vi "List Values.vi"(7 "Group":string="Default", 8 "error in (no error)":errorcluster, 9 "NI Specific Type":T2, 10 "Broad Types":T1, 11 "Blackboard in":refnum<class "Blackboard.lvclass">) -> (0 "error out":errorcluster, 1 "Values":refnum<class "Abs_Value.lvclass">[](array[class]), 2 "Tags":string[](array[string]), 3 "Blackboard out":refnum<class "Blackboard.lvclass">)   [LabVIEW 2021, in "Blackboard.lvclass"]
uses:
  Blackboard.lvclass
  <vilib>/TSA/Abstract Data Classes/Abs_Types/Value/Abs_Value.lvclass
  <vilib>/Utility/Data Type/Type Definitions/Data Type.ctl
  Support/Filter Type.ctl
  Blackboard.lvclass/Blackboard.ctl
  <vilib>/TSA/Abstract Data Classes/Abs_Types/Boolean/Abs_Boolean.lvclass
  C:/Program Files (x86)/National Instruments/LabVIEW 2021/vi.lib/TSA/Abstract Data Classes/Abs_Types/Value/Abs_Value.lvclass
  <vilib>/TSA/Abstract Data Classes/Abs_Types/String/Abs_String.lvclass
  <vilib>/TSA/Abstract Data Classes/Abs_Types/Numeric/Abs_Numeric.lvclass
  <vilib>/TSA/Abstract Data Classes/Abs_Types/Floating Point/Abs_Floating Point.lvclass
  <vilib>/TSA/Abstract Data Classes/Abs_Types/Integer/Abs_Integer.lvclass
  <vilib>/TSA/Omni-Bus/Local Bus/Support/Initialise DVR's.vi
  <vilib>/TSA/Abstract Data Classes/Abs_Types/Type/Abs_Type.lvclass
  <vilib>/Utility/Data Type/NI_Data Type.lvlib
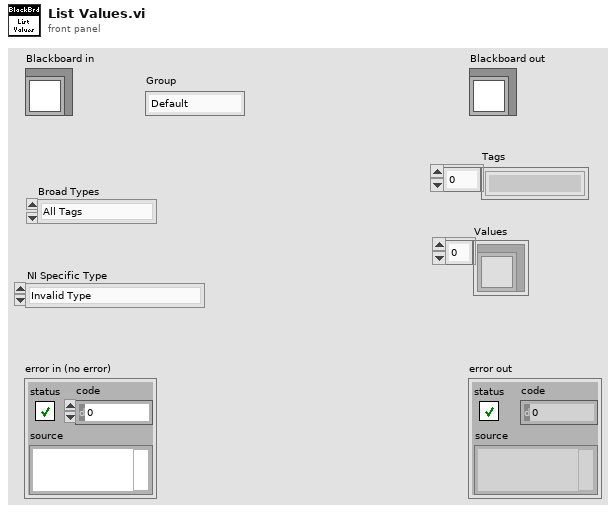
[diagram p1: front panel]
types:
  T1 = typedef "Blackboard.lvclass/Filter Type.ctl" = enum16{"All Tags", "NI Specific Type", "Boolean", "String", "Numeric", "Float", "Integer"}
  T2 = typedef "NI_Data Type.lvlib/Data Type.ctl" = enum8{"Invalid Type", "Void", "I8", "I16", "I32", "I64", "U8", "U16", "U32", "U64", "Single Float", "Double Float", "Extended Float", "Single Complex", "Double Complex", "Extended Complex", "Enum U8", "Enum U16", "Enum U32", "Enum U64", "Single Float With Unit", "Double Float With Unit", "Extended Float With Unit", "Single Complex with Unit", "Double Complex with Unit", "Extended Complex with Unit", "Boolean", "String", "Path", "Picture", "Tag", "Array", "Cluster", "Variant", "LV Variant", "Waveform", "Timestamp", "Digital Waveform", "Digital Data", "ExpressData", "Refnum", "External Data", "VI", "Poly VI", "LabVIEW Class Instance", "Fixed Point", "Set Collection", "Map Collection"}
  T3 = typedef "Blackboard.lvclass/Groups Type.ctl" = cluster{"Data":T4[], "Map":T7}
  T4 = typedef "Blackboard.lvclass/Data DVR Type.ctl" = cluster{"Tags":T5, "Data Refs":T6}
  T5 = typedef "Blackboard.lvclass/Tags Map Type.ctl" = map{string, refnum<class "Abs_Value.lvclass">}
  T6 = typedef "Local Bus.lvclass/Data Value References.ctl" = cluster{"Boolean":refnum<data-value>, "String":refnum<data-value>, "DBL":refnum<data-value>, "SGL":refnum<data-value>, "EXT":refnum<data-value>, "U8":refnum<data-value>, "U16":refnum<data-value>, "U32":refnum<data-value>, "U64":refnum<data-value>, "I8":refnum<data-value>, "I16":refnum<data-value>, "I32":refnum<data-value>, "I64":refnum<data-value>, "CDBL":refnum<data-value>, "CSGL":refnum<data-value>, "CEXT":refnum<data-value>, "Time":refnum<data-value>, "Variant":refnum<data-value>, "Waveform":refnum<data-value>, "Type":refnum<data-value>}
  T7 = typedef "Blackboard.lvclass/Group Map Type.ctl" = map{string, i32}
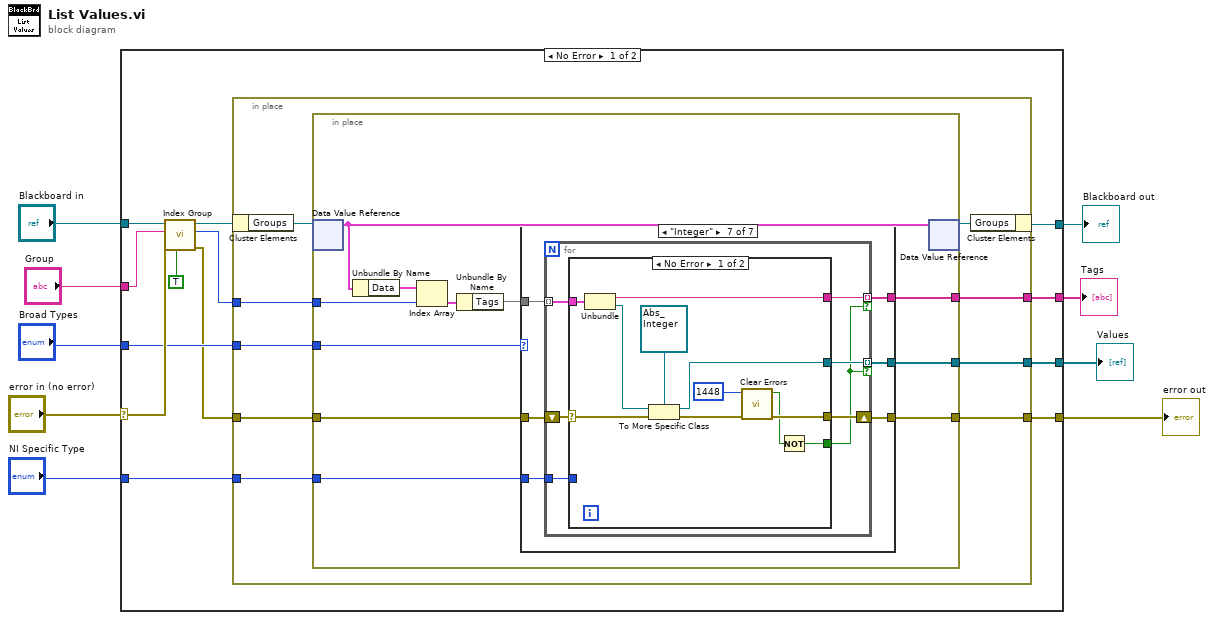
[diagram p0: block diagram]
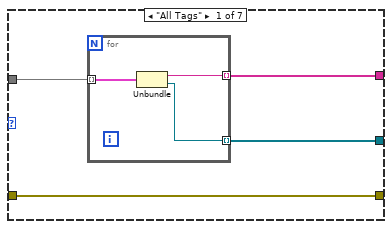
[diagram p2: hidden frame]
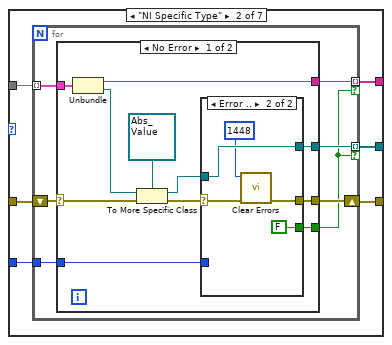
[diagram p3: hidden frame]
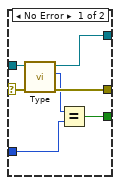
[diagram p4: hidden frame]
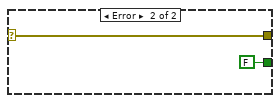
[diagram p5: hidden frame]
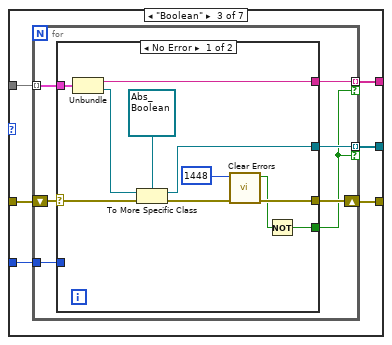
[diagram p6: hidden frame]
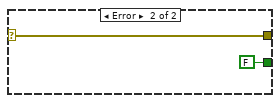
[diagram p7: hidden frame]
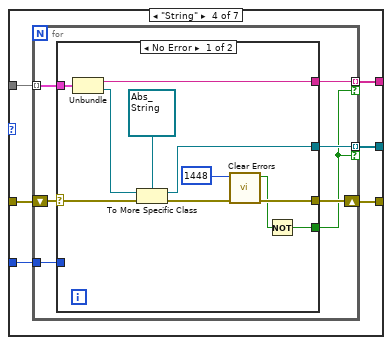
[diagram p8: hidden frame]
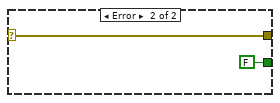
[diagram p9: hidden frame]
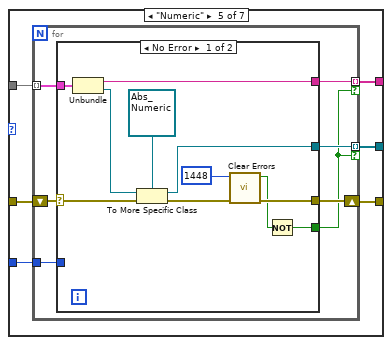
[diagram p10: hidden frame]
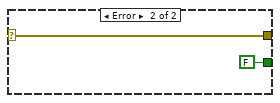
[diagram p11: hidden frame]
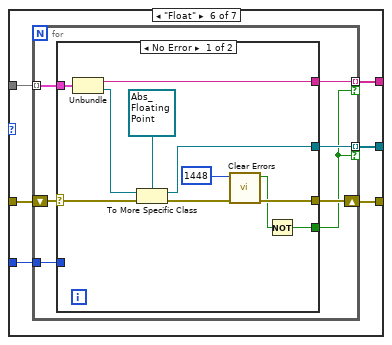
[diagram p12: hidden frame]
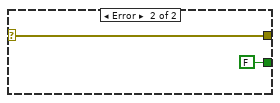
[diagram p13: hidden frame]
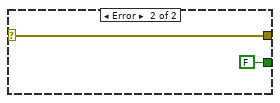
[diagram p14: hidden frame]
diagram:
  n1 = case shown="No Error" "error in (no error)" {
    selector: "error in (no error)" -> [w17 w219]
    tunnel: [w11 w219] -> w8
    tunnel: [w22 w218] -> w6
    tunnel: "Blackboard in" -> [w19 w218]
    tunnel: [w21 _] -> w5
    tunnel: [w20 _] -> w4
    tunnel: "Group" -> [w16 _]
    tunnel: "Broad Types" -> [w13 _]
    tunnel: "NI Specific Type" -> [w10 _]
    frame No Error {
      n2 = call "Index Group.vi"("Don't Create"=TRUE, "error in (no error)"=w17, "Group"=w16, "bt_Blackboard in"=w19) -> ("error out"=w12:errorcluster, "Index"=w14:i32, "bt_Blackboard out"=w18:refnum<class "Blackboard.lvclass">)  [unwired: 5 in]
      n3 = in-place {
        in-place-border: [w29] -> w21
        in-place-border: [w28] -> w20
        in-place-border: w14 -> [w27]
        in-place-border: w13 -> [w26]
        in-place-border: w12 -> [w25]
        in-place-border: [w24] -> w11
        in-place-border: w10 -> [w23]
        n4 = in-place-cluster #1(w18) -> ("Groups"=w31:refnum<data-value>)
        n5 = in-place {
          in-place-border: [w40] -> w29
          in-place-border: [w39] -> w28
          in-place-border: w27 -> [w36]
          in-place-border: w26 -> [w35]
          in-place-border: w25 -> [w34]
          in-place-border: [w33] -> w24
          in-place-border: w23 -> [w32]
          n6 = in-place-dvr #2(w31) -> (w42:T3)  [unwired: 1 out]
          n7 = Unbundle By Name(w42) -> ("Data"=w41:T4[])
          n8 = Index Array(array=w41, index=w36) -> (element=w37:T4)
          n9 = Unbundle By Name(w37) -> ("Tags"=w38:T5)
          n10 = case shown="\"Integer\"" w35 {
            tunnel: [w46 w55 w93 w119 w145 w171 w197] -> w40
            tunnel: [w45 w54 w92 w118 w144 w170 w196] -> w39
            tunnel: w38 -> [w44 w53 w91 w117 w143 w169 w195]
            tunnel: w34 -> [w43 w52 w90 w116 w142 w168 w194]
            tunnel: [w43 w51 w89 w115 w141 w167 w193] -> w33
            tunnel: w32 -> [_ w50 w88 w114 w140 w166 w192]
            frame "All Tags" {
              n11 = for {
                tunnel: w44 -> [w49] mode=indexing
                tunnel: [w48] -> w46 mode=indexing
                tunnel: [w47] -> w45 mode=indexing
                n12 = Unbundle(w49) -> (w47:string, "Value"=w48:refnum<class "Abs_Value.lvclass">)
              }
            }
            frame "NI Specific Type" {
              n13 = for {
                tunnel: w53 -> [w62] mode=indexing
                tunnel: [w60] -> w55 mode=indexing if=w56
                tunnel: [w61] -> w54 mode=indexing if=w56
                shift-right: [w58] -> w51
                shift-left: w52 -> [w59]
                tunnel: w50 -> [w57]
                n14 = case shown="No Error" w59 {
                  selector: w59 -> [w66 w87]
                  tunnel: w62 -> [w73 _]
                  tunnel: [w72 _] -> w61
                  tunnel: [w71 _] -> w60
                  tunnel: [w65 w87] -> w58
                  tunnel: w57 -> [w64 _]
                  tunnel: [w63 FALSE] -> w56
                  frame No Error {
                    n15 = Unbundle(w73) -> (w72:string, "Value"=w67:refnum<class "Abs_Value.lvclass">)
                    n16 = To More Specific Class(target class=refnum<class "Abs_Value.lvclass"> refnum ("Abs_Value.lvclass"), reference=w67, error in=w66) -> (specific class reference=w68:refnum<class "Abs_Value.lvclass">, error out=w69:errorcluster)
                    n17 = case shown="Error .." w69 {
                      selector: w69 -> [w79 w83]
                      tunnel: [w80 w85] -> w71
                      tunnel: w68 -> [w78 w85]
                      tunnel: [w77 w82] -> w65
                      tunnel: w64 -> [w75 _]
                      tunnel: [w74 FALSE] -> w63
                      frame No Error {
                        n18 = call-dynamic "Type.vi"("error in (no error)"=w79, "Element in"=w78) -> ("error out"=w77:errorcluster, "Type"=w76:T2, "Element out"=w80:refnum<class "Abs_Value.lvclass">)  [unwired: 7 in]
                        n19 = Equal?(x=w76, y=w75) -> (x = y?=w74:bool)
                      }
                      frame Error {
                        n20 = call <vilib>:"Clear Errors.vi"("error in (no error)"=w83, "specific error code to clear (0: all)"=1448) -> ("error out"=w82:errorcluster)  [unwired: 4 in, 1 out]
                      }
                    }
                  }
                  frame Error {
                  }
                }
              }
            }
            frame "Boolean" {
              n21 = for {
                tunnel: w91 -> [w100] mode=indexing
                tunnel: [w98] -> w93 mode=indexing if=w94
                tunnel: [w99] -> w92 mode=indexing if=w94
                shift-right: [w96] -> w89
                shift-left: w90 -> [w97]
                tunnel: w88 -> [w95]
                n22 = case shown="No Error" w97 {
                  selector: w97 -> [w106 w113]
                  tunnel: w100 -> [w111 _]
                  tunnel: [w110 _] -> w99
                  tunnel: [w108 _] -> w98
                  tunnel: [w105 w113] -> w96
                  tunnel: w95 -> [_ _]
                  tunnel: [w102 FALSE] -> w94
                  frame No Error {
                    n23 = Unbundle(w111) -> (w110:string, "Value"=w107:refnum<class "Abs_Value.lvclass">)
                    n24 = To More Specific Class(target class=refnum<class "Abs_Boolean.lvclass"> refnum ("Abs_Boolean.lvclass"), reference=w107, error in=w106) -> (specific class reference=w108:refnum<class "Abs_Boolean.lvclass">, error out=w109:errorcluster)
                    n25 = call <vilib>:"Clear Errors.vi"("error in (no error)"=w109, "specific error code to clear (0: all)"=1448) -> ("error out"=w105:errorcluster, "specific error cleared?"=w101:bool)  [unwired: 4 in]
                    n26 = Not(x=w101) -> (.not. x?=w102:bool)
                  }
                  frame Error {
                  }
                }
              }
            }
            frame "String" {
              n27 = for {
                tunnel: w117 -> [w126] mode=indexing
                tunnel: [w124] -> w119 mode=indexing if=w120
                tunnel: [w125] -> w118 mode=indexing if=w120
                shift-right: [w122] -> w115
                shift-left: w116 -> [w123]
                tunnel: w114 -> [w121]
                n28 = case shown="No Error" w123 {
                  selector: w123 -> [w132 w139]
                  tunnel: w126 -> [w137 _]
                  tunnel: [w136 _] -> w125
                  tunnel: [w134 _] -> w124
                  tunnel: [w131 w139] -> w122
                  tunnel: w121 -> [_ _]
                  tunnel: [w129 FALSE] -> w120
                  frame No Error {
                    n29 = Unbundle(w137) -> (w136:string, "Value"=w133:refnum<class "Abs_Value.lvclass">)
                    n30 = To More Specific Class(target class=refnum<class "Abs_String.lvclass"> refnum ("Abs_String.lvclass"), reference=w133, error in=w132) -> (specific class reference=w134:refnum<class "Abs_String.lvclass">, error out=w135:errorcluster)
                    n31 = call <vilib>:"Clear Errors.vi"("error in (no error)"=w135, "specific error code to clear (0: all)"=1448) -> ("error out"=w131:errorcluster, "specific error cleared?"=w128:bool)  [unwired: 4 in]
                    n32 = Not(x=w128) -> (.not. x?=w129:bool)
                  }
                  frame Error {
                  }
                }
              }
            }
            frame "Numeric" {
              n33 = for {
                tunnel: w143 -> [w152] mode=indexing
                tunnel: [w150] -> w145 mode=indexing if=w146
                tunnel: [w151] -> w144 mode=indexing if=w146
                shift-right: [w148] -> w141
                shift-left: w142 -> [w149]
                tunnel: w140 -> [w147]
                n34 = case shown="No Error" w149 {
                  selector: w149 -> [w158 w165]
                  tunnel: w152 -> [w163 _]
                  tunnel: [w162 _] -> w151
                  tunnel: [w160 _] -> w150
                  tunnel: [w157 w165] -> w148
                  tunnel: w147 -> [_ _]
                  tunnel: [w155 FALSE] -> w146
                  frame No Error {
                    n35 = Unbundle(w163) -> (w162:string, "Value"=w159:refnum<class "Abs_Value.lvclass">)
                    n36 = To More Specific Class(target class=refnum<class "Abs_Numeric.lvclass"> refnum ("Abs_Numeric.lvclass"), reference=w159, error in=w158) -> (specific class reference=w160:refnum<class "Abs_Numeric.lvclass">, error out=w161:errorcluster)
                    n37 = call <vilib>:"Clear Errors.vi"("error in (no error)"=w161, "specific error code to clear (0: all)"=1448) -> ("error out"=w157:errorcluster, "specific error cleared?"=w154:bool)  [unwired: 4 in]
                    n38 = Not(x=w154) -> (.not. x?=w155:bool)
                  }
                  frame Error {
                  }
                }
              }
            }
            frame "Float" {
              n39 = for {
                tunnel: w169 -> [w178] mode=indexing
                tunnel: [w176] -> w171 mode=indexing if=w172
                tunnel: [w177] -> w170 mode=indexing if=w172
                shift-right: [w174] -> w167
                shift-left: w168 -> [w175]
                tunnel: w166 -> [w173]
                n40 = case shown="No Error" w175 {
                  selector: w175 -> [w184 w191]
                  tunnel: w178 -> [w189 _]
                  tunnel: [w188 _] -> w177
                  tunnel: [w186 _] -> w176
                  tunnel: [w183 w191] -> w174
                  tunnel: w173 -> [_ _]
                  tunnel: [w181 FALSE] -> w172
                  frame No Error {
                    n41 = Unbundle(w189) -> (w188:string, "Value"=w185:refnum<class "Abs_Value.lvclass">)
                    n42 = To More Specific Class(target class=refnum<class "Abs_Floating Point.lvclass"> refnum ("Abs_Floating Point.lvclass"), reference=w185, error in=w184) -> (specific class reference=w186:refnum<class "Abs_Floating Point.lvclass">, error out=w187:errorcluster)
                    n43 = call <vilib>:"Clear Errors.vi"("error in (no error)"=w187, "specific error code to clear (0: all)"=1448) -> ("error out"=w183:errorcluster, "specific error cleared?"=w180:bool)  [unwired: 4 in]
                    n44 = Not(x=w180) -> (.not. x?=w181:bool)
                  }
                  frame Error {
                  }
                }
              }
            }
            frame "Integer" {
              n45 = for {
                tunnel: w195 -> [w204] mode=indexing
                tunnel: [w202] -> w197 mode=indexing if=w198
                tunnel: [w203] -> w196 mode=indexing if=w198
                shift-right: [w200] -> w193
                shift-left: w194 -> [w201]
                tunnel: w192 -> [w199]
                n46 = case shown="No Error" w201 {
                  selector: w201 -> [w210 w217]
                  tunnel: w204 -> [w215 _]
                  tunnel: [w214 _] -> w203
                  tunnel: [w212 _] -> w202
                  tunnel: [w209 w217] -> w200
                  tunnel: w199 -> [_ _]
                  tunnel: [w207 FALSE] -> w198
                  frame No Error {
                    n47 = Unbundle(w215) -> (w214:string, "Value"=w211:refnum<class "Abs_Value.lvclass">)
                    n48 = To More Specific Class(target class=refnum<class "Abs_Integer.lvclass"> refnum ("Abs_Integer.lvclass"), reference=w211, error in=w210) -> (specific class reference=w212:refnum<class "Abs_Integer.lvclass">, error out=w213:errorcluster)
                    n49 = call <vilib>:"Clear Errors.vi"("error in (no error)"=w213, "specific error code to clear (0: all)"=1448) -> ("error out"=w209:errorcluster, "specific error cleared?"=w206:bool)  [unwired: 4 in]
                    n50 = Not(x=w206) -> (.not. x?=w207:bool)
                  }
                  frame Error {
                  }
                }
              }
            }
          }
          n51 = in-place-dvr #2(w42) -> (w30:refnum<data-value>)  [unwired: 1 out]
        }
        n52 = in-place-cluster #1("Groups"=w30) -> (w22:refnum<class "Blackboard.lvclass">)
      }
    }
    frame Error {
    }
  }
  "error out" <- w8
  "Blackboard out" <- w6
  "Values" <- w5
  "Tags" <- w4
